vi "ScaleData(Scalar).vi"(5 "Offset":dbl, 7 "Factor":dbl, 11 "Data in":dbl) -> (3 "Data out":dbl)   [LabVIEW 2014]
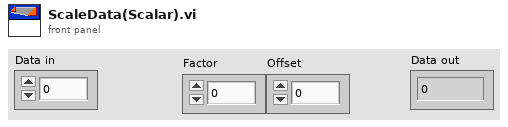
[diagram p1: front panel]
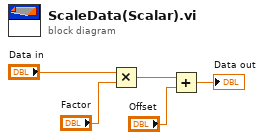
[diagram p0: block diagram]
diagram:
  n1 = Multiply(x="Data in", y="Factor") -> (x*y=w5:dbl)
  n2 = Add(x=w5, y="Offset") -> (x+y=→"Data out":dbl)
